vi "Algo3.vi"(0 "Range (Threshold 1)":cluster{"Lower value":sgl, "Upper value":sgl}={"Lower value"=0.0, "Upper value"=47.0}, 7 "error in":errorcluster) -> (20 "Circles (Shape Detection 1)":T2(array[cluster]) {"Position"."Y" format="%.2f"; "Position"."X" format="%.2f"}, 22 "Number of Matches (Shape Detection 1)":i32, 27 "error out":errorcluster)   [LabVIEW 2015]
uses:
  <vilib>/vision/NI_Vision_Development_Module.lvlib
panel:
  in  "Radius":sgl
  out "Cycle Timing":u32
  in  "stop":bool
  out "Image Out":T1(plugin-control)
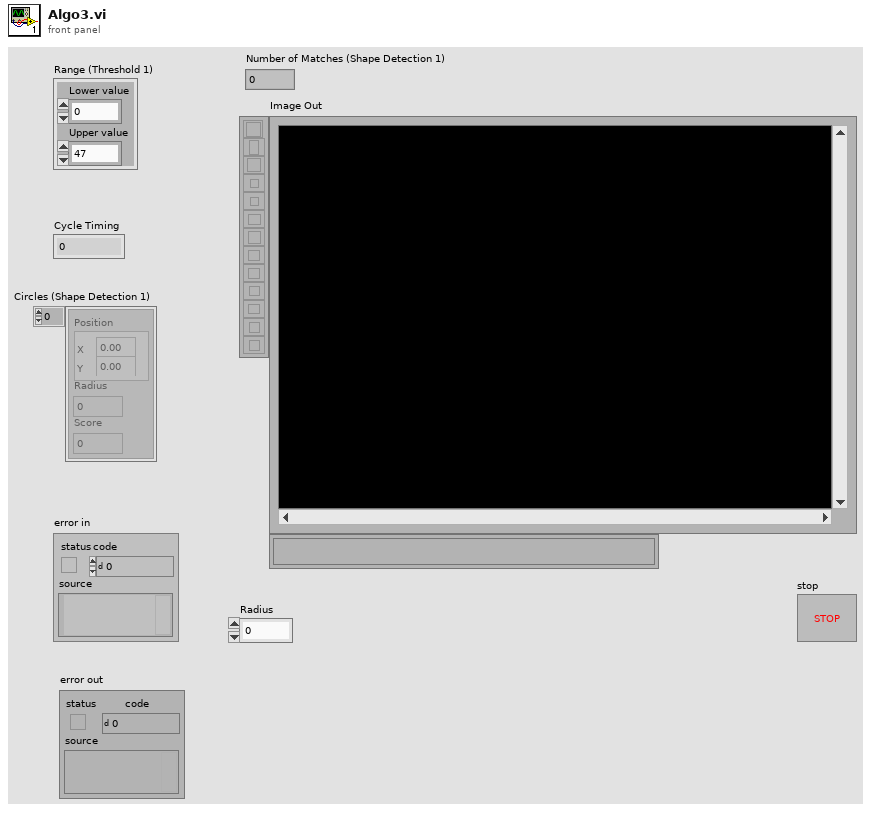
[diagram p1: front panel]
types:
  T1 = typedef "IMAQ Image.ctl" = refnum<image>
  T2 = cluster{"Position":cluster{"X":sgl, "Y":sgl}, "Radius":dbl, "Score":dbl}[]
  T3 = typedef "Image Type" = u32
  T4 = cluster{"Left":i32, "Top":i32, "Right":i32, "Bottom":i32}
  T5 = cluster{"Extraction Mode":u32, "Edge Threshold":i32, "Edge Filter Size":u32, "Min Length":i32, "Row Search Step Size":i32, "Col Search Step Size":i32, "Max Endpoint Gap":i32, "Closed":bool, "Subpixel":bool}
  T6 = cluster{"Rotation":bool, "Scale":bool, "Occlusion":bool, "Range Settings":cluster{"Match Constraints":u32, "Min":dbl, "Max":dbl}[]}
  T7 = cluster{"Global Rectangle":i32[], "Contours":cluster{"ID":enum32{"External", "Internal"}, "Type":u32, "Coordinates":i32[]}[]}
  T8 = cluster{"Position":cluster{"X":sgl, "Y":sgl}, "Radius":dbl, "Score":dbl}
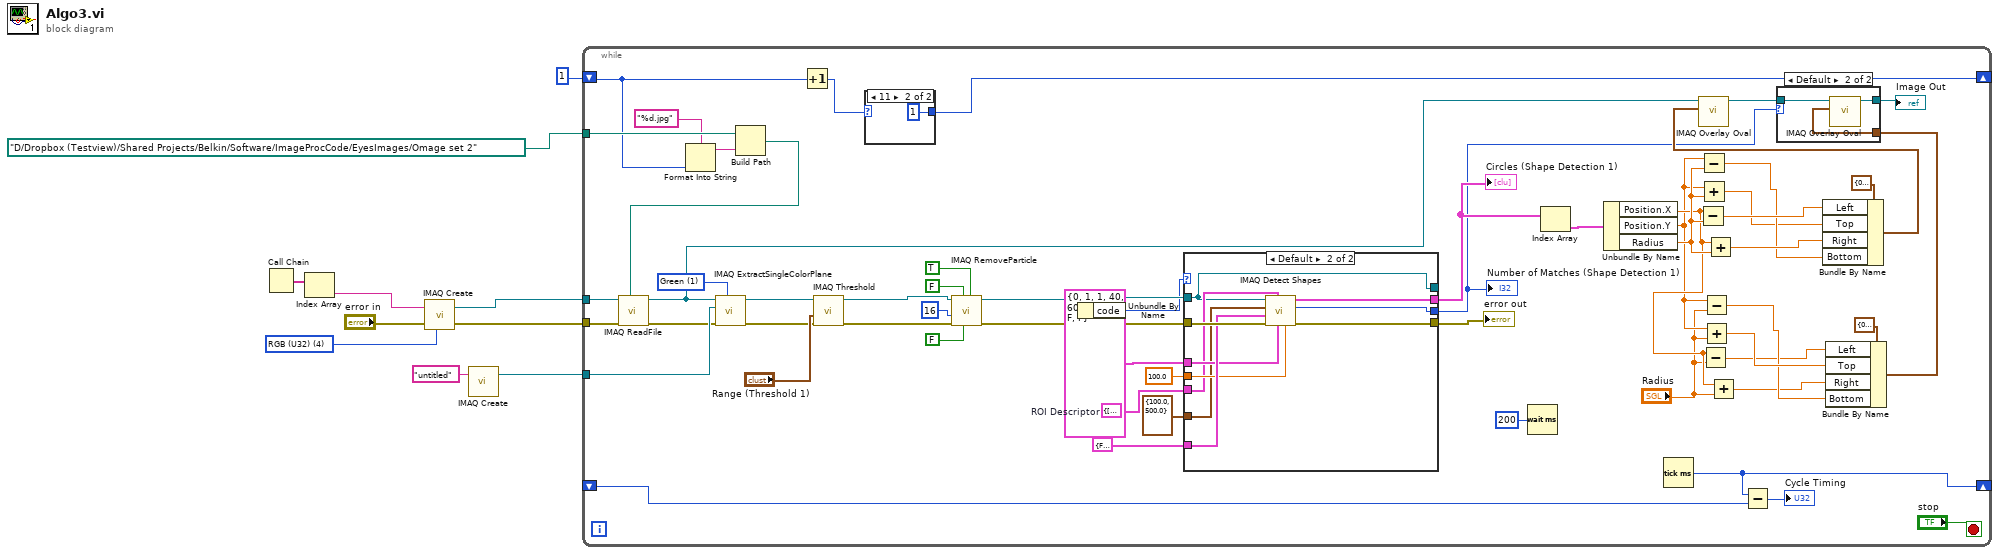
[diagram p0: block diagram]
diagram:
  w7 = T3 4 items=["Grayscale (U8)", "Grayscale (I16)", "Grayscale (SGL)", "Complex (CSG)", "RGB (U32)", "HSL (U32)", "RGB (U64)", "Grayscale (U16)"] ("Image Type")
  n1 = Call Chain() -> (call chain=w9:string[])
  n2 = Index Array(array=w9) -> (element=w8:string)  [unwired: 1 in]
  n3 = call "IMAQ Create"("Image Name"=w8, "Image Type"=w7, "error in (no error)"="error in") -> ("New Image"=w4:T1, "error out"=w3:errorcluster)  [unwired: 1 in, 1 out]
  n4 = call "IMAQ Create"("Image Name"="untitled") -> ("New Image"=w5:T1)  [unwired: 3 in, 2 out]
  n5 = while {
    tunnel: w3 -> [w33]
    tunnel: w5 -> [w49]
    tunnel: w4 -> [w34]
    shift-right: [w37] -> _
    shift-left: _ -> [w36]
    shift-right: [w29] -> _
    shift-left: 1 -> [w25]
    tunnel: path "D:/Dropbox (Testview)/Shared Projects/Belkin/Software/ImageProcCode/EyesImages/Omage set 2" -> [w28]
    stop <- "stop" stop-if-true
    w53 = T7 {"Global Rectangle"=[20, 20, 1580, 1024], "Contours"=[{"ID"=enum."External", "Type"=3, "Coordinates"=[20, 20, 1580, 1024]}]}  # ROI Descriptor
    w67 = 1 items=["Red", "Green", "Blue", "Hue", "Saturation", "Luminance", "Value", "Intensity"] ("Color Plane")
    n6 = Format Into String(format string="%d.jpg", w25) -> (resulting string=w27:string)  [unwired: 2 in, 1 out]
    n7 = Build Path(base path=w28, name or relative path=w27) -> (appended path=w24:path)
    n8 = call "IMAQ ReadFile"("File Path"=w24, "error in (no error)"=w33, "Image"=w34) -> ("error out"=w32:errorcluster, "Image Out"=w31:T1)  [unwired: 2 in, 5 out]
    n9 = call "IMAQ ExtractSingleColorPlane"("Color Plane"=w67, "error in (no error)"=w32, "Image Dst"=w49, "Image Src"=w31) -> ("error out"=w64:errorcluster, "Image Dst Out"=w65:T1)  [unwired: 6 out]
    n10 = Increment(x=w25) -> (x+1=w30:i32)
    n11 = call "IMAQ Threshold"("error in (no error)"=w64, "Range"="Range (Threshold 1)", "Image Src"=w65) -> ("error out"=w58:errorcluster, "Image Dst Out"=w59:T1)  [unwired: 3 in, 4 out]
    n12 = case shown="11" w30 {
      selector: w30 -> [w72 _]
      tunnel: [w72 1] -> w29
      frame 0, Default {
      }
      frame 11 {
      }
    }
    n13 = call "IMAQ RemoveParticle"("Connectivity 4/8 (8)"=TRUE, "Low Pass/High Pass (Low)"=FALSE, "Square/Hexa (Square)"=FALSE, "error in (no error)"=w58, "Number of Erosion"=16, "Image Src"=w59) -> ("error out"=w51:errorcluster, "Image Dst Out"=w52:T1)  [unwired: 1 in, 3 out]
    n14 = Unbundle By Name(w51) -> ("code"=w50:i32)
    n15 = case shown="Default" w50 {
      tunnel: w51 -> [_ w84]
      tunnel: [_ w83] -> w11
      tunnel: T6 {"Rotation"=FALSE, "Scale"=FALSE, "Occlusion"=TRUE, "Range Settings"=[{"Match Constraints"=2, "Min"=0.0, "Max"=50.0}]} ("Match Options") -> [_ w82]
      tunnel: T5 {"Extraction Mode"=0, "Edge Threshold"=1, "Edge Filter Size"=1, "Min Length"=40, "Row Search Step Size"=60, "Col Search Step Size"=60, "Max Endpoint Gap"=10, "Closed"=FALSE, "Subpixel"=FALSE} ("Curve Parameters") -> [_ w81]
      tunnel: 100.0 ("Minimum match score") -> [_ w80]
      tunnel: cluster{"Min Radius":dbl, "Max Radius":dbl} {"Min Radius"=100.0, "Max Radius"=500.0} ("Circle Descriptor") -> [_ w79]
      tunnel: w53 -> [_ w78]
      tunnel: [_ w77] -> w46
      tunnel: w52 -> [w74 w75]
      tunnel: [_ w76] -> w48
      tunnel: [w74 w75] -> _
      frame -1074396199, -1074396198 {
        # "Discard Coordinate\nSystem Error"
      }
      frame Default {
        n16 = call-poly "IMAQ Detect Shapes"("Minimum match score"=w80, "Curve Parameters"=w81, "ROI Descriptor"=w78, "error in (no error)"=w84, "Match Options"=w82, "Circle Descriptor"=w79, "Image"=w75) -> ("error out"=w76:errorcluster, "Number of Matches Returned"=w83:i32, "Circles"=w77:T2)  [unwired: 2 out]
      }
    }
    "Number of Matches (Shape Detection 1)" <- w11
    "Circles (Shape Detection 1)" <- w46
    "error out" <- w48
    n17 = Wait (ms)(milliseconds to wait=u32 200) -> ()  [unwired: 1 out]
    n18 = Index Array(array=w46) -> (element=w45:T8)  [unwired: 1 in]
    n19 = Unbundle By Name(w45) -> ("Position.X"=w15:sgl, "Position.Y"=w14:sgl, "Radius"=w42:dbl)
    n20 = Tick Count (ms)() -> (millisecond timer value=w37:u32)
    n21 = Subtract(x=w15, y=w42) -> (x-y=w44:dbl)
    n22 = Subtract(x=w14, y=w42) -> (x-y=w41:dbl)
    n23 = Add(x=w14, y=w42) -> (x+y=w40:dbl)
    n24 = Subtract(x=w15, y="Radius") -> (x-y=w17:sgl)
    n25 = Subtract(x=w14, y="Radius") -> (x-y=w19:sgl)
    n26 = Add(x=w14, y="Radius") -> (x+y=w20:sgl)
    n27 = Add(x=w15, y=w42) -> (x+y=w43:dbl)
    n28 = Add(x=w15, y="Radius") -> (x+y=w18:sgl)
    n29 = Subtract(x=w37, y=w36) -> (x-y=→"Cycle Timing":u32)
    n30 = Bundle By Name(cluster=T4 {"Left"=0, "Top"=0, "Right"=0, "Bottom"=0} ("Bounding Rectangle"), "Left"=w44, "Top"=w40, "Right"=w43, "Bottom"=w41) -> (w39:T4)
    n31 = call "IMAQ Overlay Oval"("Bounding Rectangle"=w39, "Image"=w31) -> ("Image Out"=w22:T1)  [unwired: 8 in, 1 out]
    n32 = Bundle By Name(cluster=T4 {"Left"=0, "Top"=0, "Right"=0, "Bottom"=0} ("Bounding Rectangle"), "Left"=w17, "Top"=w20, "Right"=w18, "Bottom"=w19) -> (w12:T4)
    n33 = case shown="Default" w11 {
      tunnel: w22 -> [w68 w71]
      tunnel: [w68 w70] -> w21
      tunnel: w12 -> [_ w69]
      frame 0 {
      }
      frame Default {
        n34 = call "IMAQ Overlay Oval"("Bounding Rectangle"=w69, "Image"=w71) -> ("Image Out"=w70:T1)  [unwired: 8 in, 1 out]
      }
    }
    "Image Out" <- w21
  }
